vi "updateToVersion.vi"(8 "error in (no error)":errorcluster, 10 "Version":string, 11 "hgHandler in":refnum<class "hgHandler.lvclass">) -> (0 "error out":errorcluster, 1 "Log":string, 3 "hgHandler out":refnum<class "hgHandler.lvclass">)   [LabVIEW 2013, in "hgHandler.lvclass"]
uses:
  hgHandler.lvclass
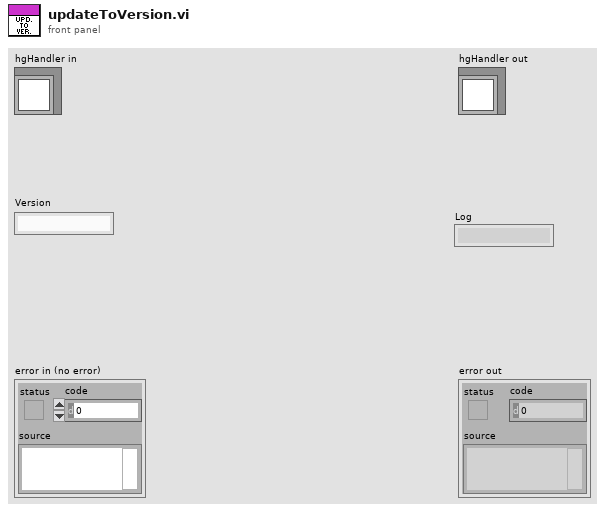
[diagram p1: front panel]
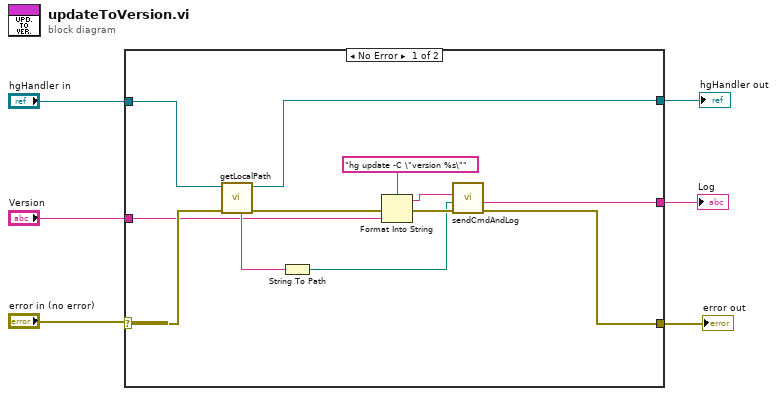
[diagram p0: block diagram]
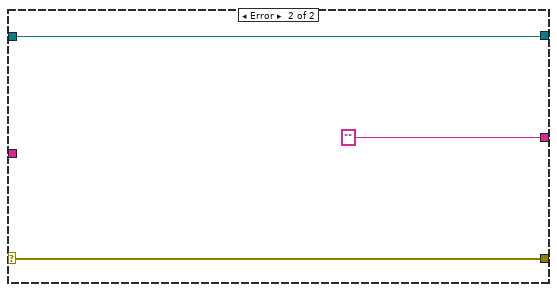
[diagram p2: hidden frame]
diagram:
  n1 = case shown="No Error" "error in (no error)" {
    selector: "error in (no error)" -> [w17 w21]
    tunnel: "hgHandler in" -> [w18 w20]
    tunnel: [w14 w21] -> w4
    tunnel: "Version" -> [w7 _]
    tunnel: [w9 "" ("Log")] -> w1
    tunnel: [w8 w20] -> w2
    frame No Error {
      n2 = call-dynamic "getLocalPath.vi"("error in (no error)"=w17, "repoHandler in"=w18) -> ("error out"=w13:errorcluster, "repoHandler out"=w8:refnum<class "hgHandler.lvclass">, "Local Path"=w15:string)  [unwired: 7 in]
      n3 = String To Path(string=w15) -> (path=w11:path)
      n4 = Format Into String(format string="hg update -C \"version %s\"", error in=w13, w7) -> (resulting string=w10:string, error out=w12:errorcluster)  [unwired: 1 in]
      n5 = call "sendCmdAndLog.vi"("error in (no error)"=w12, "working directory"=w11, "command"=w10) -> ("error out"=w14:errorcluster, "Log"=w9:string)  [unwired: 6 in, 1 out]
    }
    frame Error {
    }
  }
  "error out" <- w4
  "hgHandler out" <- w2
  "Log" <- w1
